vi "Read Device Information.vi"(8 "error in (no error)":errorcluster, 11 "Controller in":refnum<class "Controller.lvclass">) -> (0 "error out":errorcluster, 2 "Device Information":T1 {"Product ID" format="%.0x"}, 3 "Controller out":refnum<class "Controller.lvclass">)   [LabVIEW 2015, in "SMI.lvlib" / "Controller.lvclass"]
uses:
  Controller.lvclass
  Controls/DeviceInformation.ctl
  Controller.lvclass/Controller.ctl
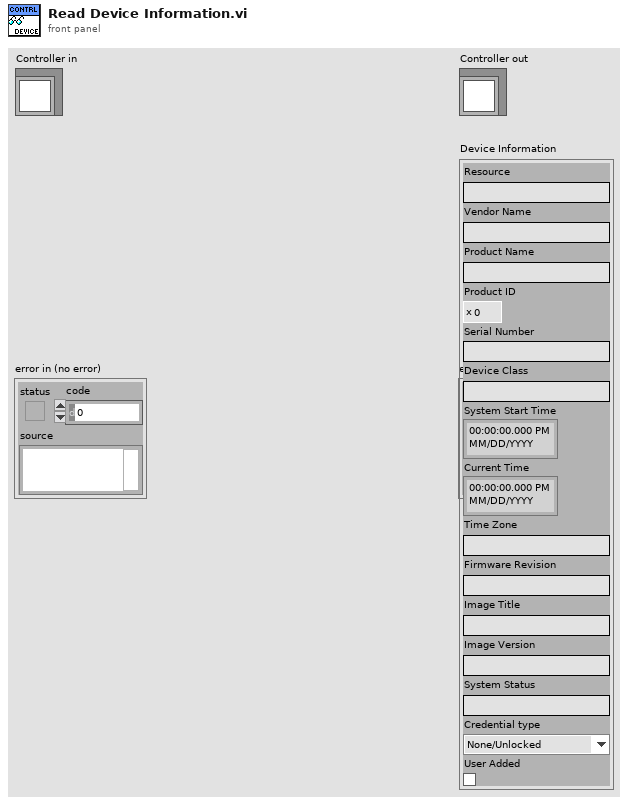
[diagram p1: front panel]
types:
  T1 = typedef "SMI.lvlib/Controller.lvclass/DeviceInformation.ctl" = cluster{"Resource":string, "Vendor Name":string, "Product Name":string, "Product ID":u32, "Serial Number":string, "Device Class":string, "System Start Time":timestamp, "Current Time":timestamp, "Time Zone":string, "Firmware Revision":string, "Image Title":string, "Image Version":string, "System Status":string, "Credential type":enum16{"None/Unlocked", "FTP Password", "NIAuth Credentials"}, "User Added":bool}
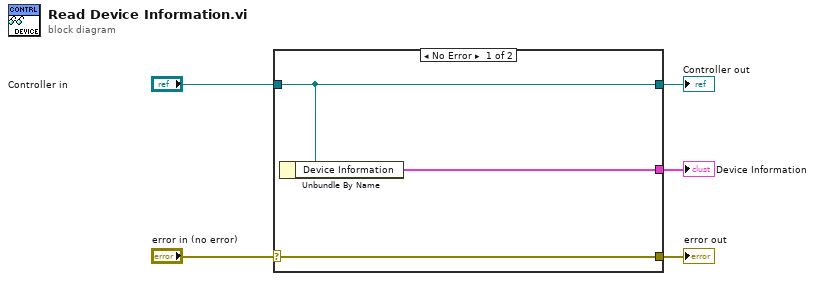
[diagram p0: block diagram]
diagram:
  n1 = case shown="No Error" "error in (no error)" {
    selector: "error in (no error)" -> [w8 w9]
    tunnel: [w8 w9] -> w4
    tunnel: [w7 w10] -> w2
    tunnel: "Controller in" -> [w7 w10]
    tunnel: [w6 _] -> w1
    frame No Error {
      n2 = Unbundle By Name(w7) -> ("Device Information"=w6:T1)
    }
    frame Error {
    }
  }
  "error out" <- w4
  "Controller out" <- w2
  "Device Information" <- w1
